vi "slider_connection.vi"(6 "2*g":dbl, 7 "A (Crosssection of Tank 1)\n[m²]":dbl, 8 "a1":dbl, 9 "outflow":dbl, 10 "Slide Refnum in":refnum<vi>, 11 "Slide in":refnum<vi>) -> ()   [LabVIEW 2020]
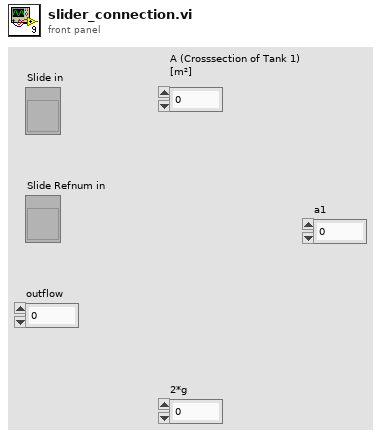
[diagram p1: front panel]
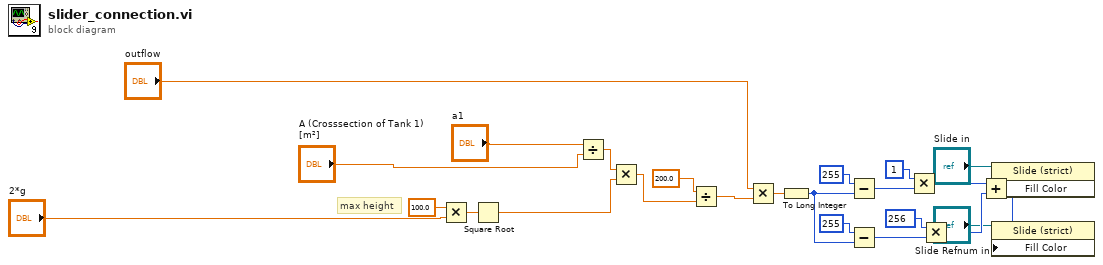
[diagram p0: block diagram]
diagram:
  # "max height"
  n1 = Multiply(x=100.0 ("y"), y="2*g") -> (x*y=w22:dbl)
  n2 = Square Root(x=w22) -> (sqrt(x)=w1:dbl)
  n3 = Divide(x="a1", y="A (Crosssection of Tank 1)\n[m²]") -> (x/y=w3:dbl)
  n4 = Multiply(x=w3, y=w1) -> (x*y=w2:dbl)
  n5 = Divide(x=200.0, y=w2) -> (x/y=w19:dbl)
  n6 = Multiply(x="outflow", y=w19) -> (x*y=w8:dbl)
  n7 = To Long Integer(number=w8) -> (32bit integer=w16:i32)
  n8 = Subtract(x=255, y=w16) -> (x-y=w14:i32)
  n9 = Subtract(x=255, y=w16) -> (x-y=w17:i32)
  n10 = Multiply(x=1, y=w14) -> (x*y=w9:i32)
  n11 = Multiply(x=256, y=w17) -> (x*y=w10:i32)
  n12 = Add(x=w9, y=w10) -> (x+y=w23:i32)
  n13 = property on="Property Node" class="Slide (strict)"(reference="Slide in", "Fill Color"=w23) -> ()  [unwired: 1 in, 2 out]
  n14 = property on="Property Node" class="Slide (strict)"(reference="Slide Refnum in", "Fill Color"=w23) -> ()  [unwired: 1 in, 2 out]
